vi "LVDT Setting.vi"(8 "error in (no error)":errorcluster) -> (0 "error out 2":errorcluster)   [LabVIEW 2015]
uses:
  Control Button/Save.ctl
  Control Button/Exit.ctl
  Control Button/Delete.ctl
  <vilib>/addons/database/Connection.llb/DB Tools Open Connec (String).vi
  <vilib>/addons/database/_DB Variant To Data/Database Variant To Data.xnode
  <vilib>/addons/database/NI_Database_API.lvlib
panel:
  in  "Delete":T1
  out "data":string[](array[string])
  out "Model change":string
  in  "Model Select":string(combo)
  out "error out":errorcluster
  in  "Exit":T2
  in  "Save":T3
  in  "Sensor Setting Data":T4 {"LVDT4Max(mm) AI3" format="%0.02f"; "LVDT3Max(mm) AI2" format="%0.02f"; "LVDT2Max(mm) AI1" format="%0.02f"; "LVDT1Max(mm) AI0" format="%0.02f"; "LVDT4Min(mm) AI3" format="%0.02f"; "LVDT3Min(mm) AI2" format="%0.02f"; "LVDT2Min(mm) AI1" format="%0.02f"; "LVDT1Min (mm)AI0" format="%0.02f"}
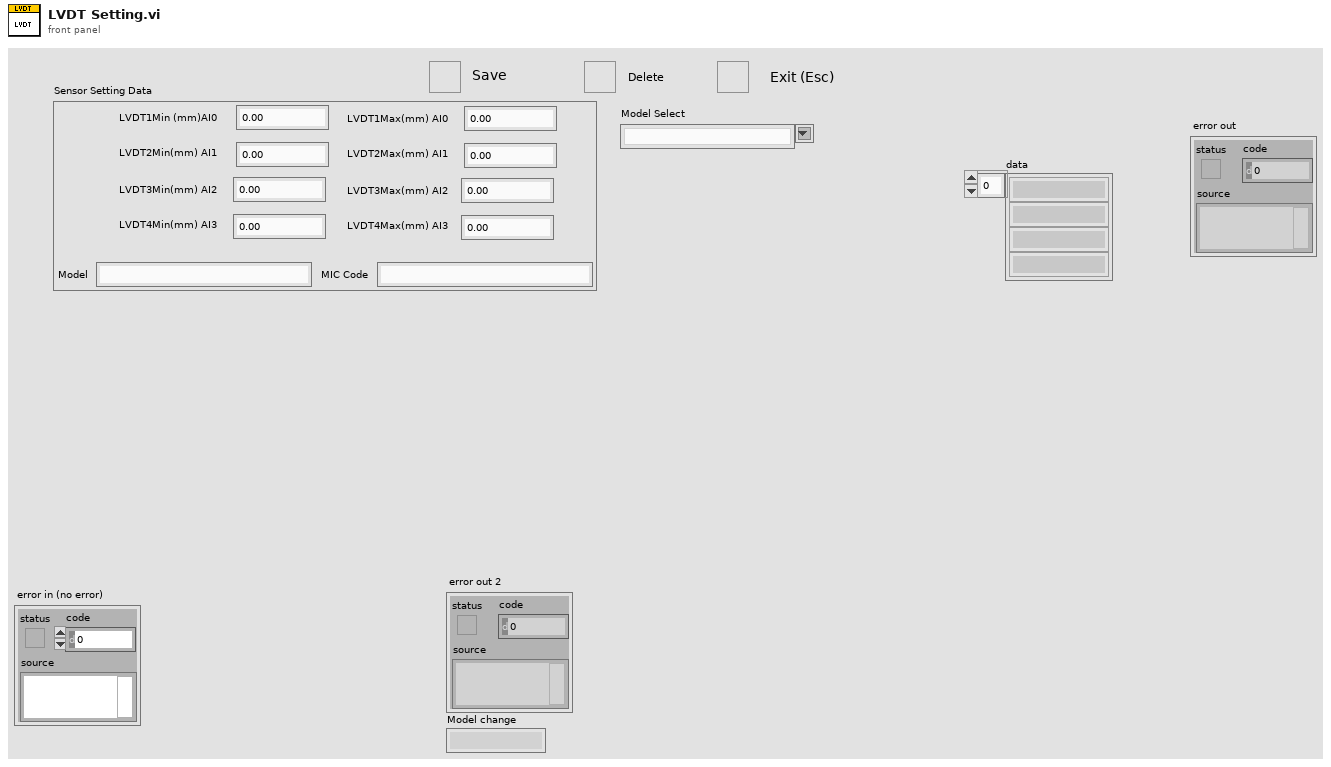
[diagram p1: front panel]
types:
  T1 = typedef "Delete.ctl" = bool
  T2 = typedef "Exit.ctl" = bool
  T3 = typedef "Save.ctl" = bool
  T4 = cluster{"LVDT1Max(mm) AI0":dbl, "LVDT1Min (mm)AI0":dbl, "LVDT2Max(mm) AI1":dbl, "LVDT2Min(mm) AI1":dbl, "LVDT3Max(mm) AI2":dbl, "LVDT3Min(mm) AI2":dbl, "LVDT4Max(mm) AI3":dbl, "LVDT4Min(mm) AI3":dbl, "Model":string, "MIC Code":string}
  T5 = typedef "NI_Database_API.lvlib/Conn ObjectReference.ctl" = refnum<k1>
  T6 = enum16{"Left Button", "Center Button", "Right Button", "Window Close"}
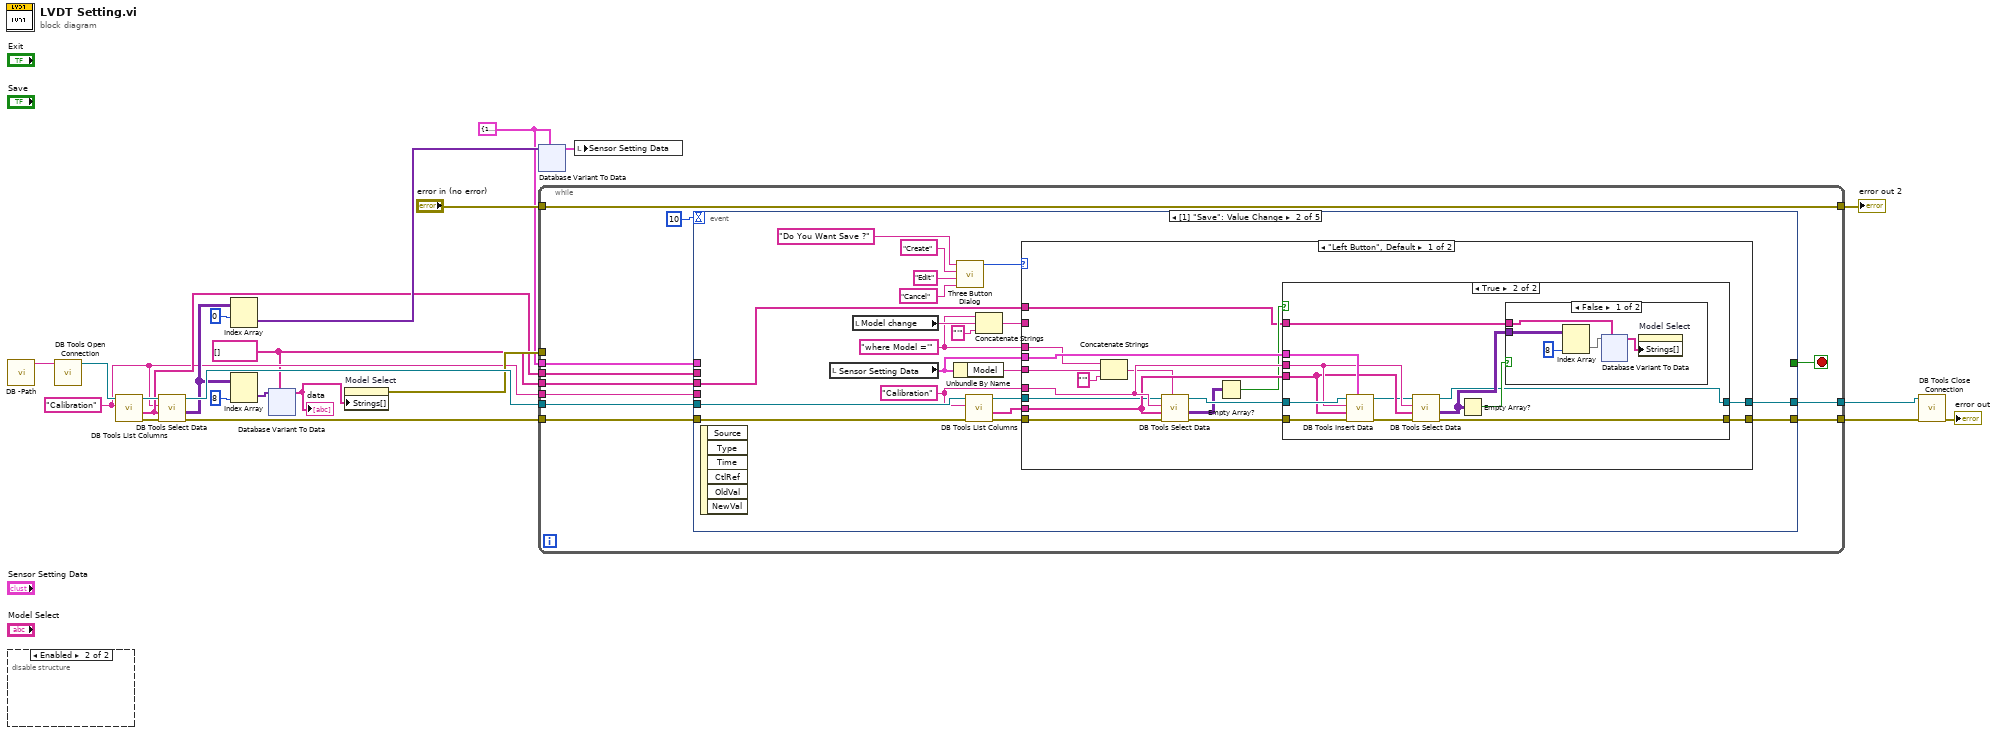
[diagram p0: block diagram]
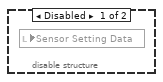
[diagram p2: hidden frame]
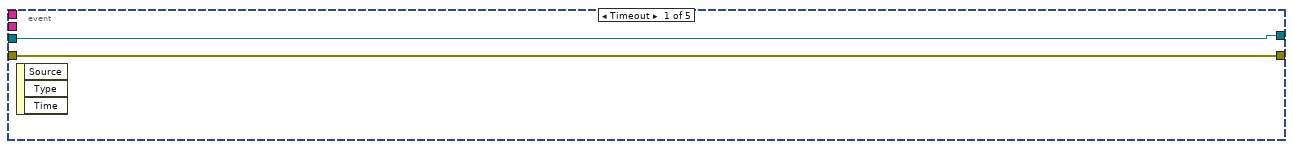
[diagram p3: hidden frame]
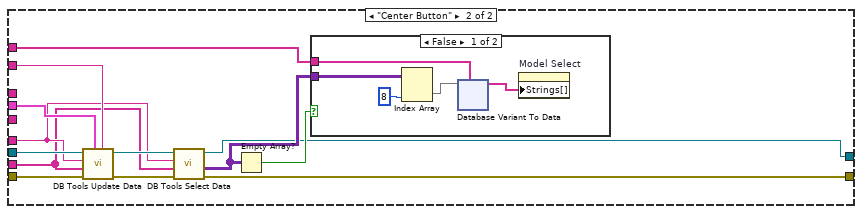
[diagram p6: hidden frame]
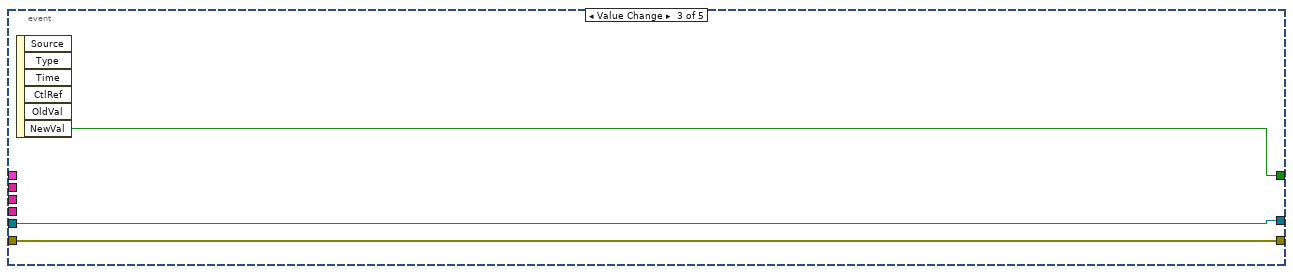
[diagram p8: hidden frame]
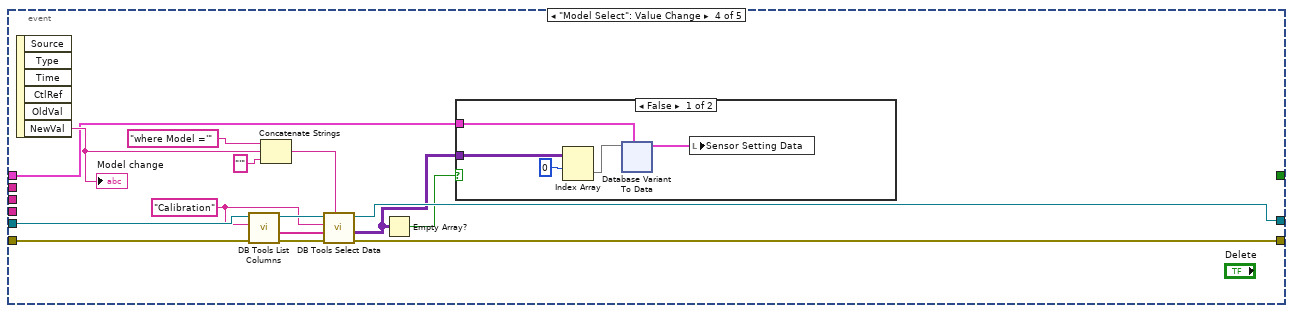
[diagram p9: hidden frame]
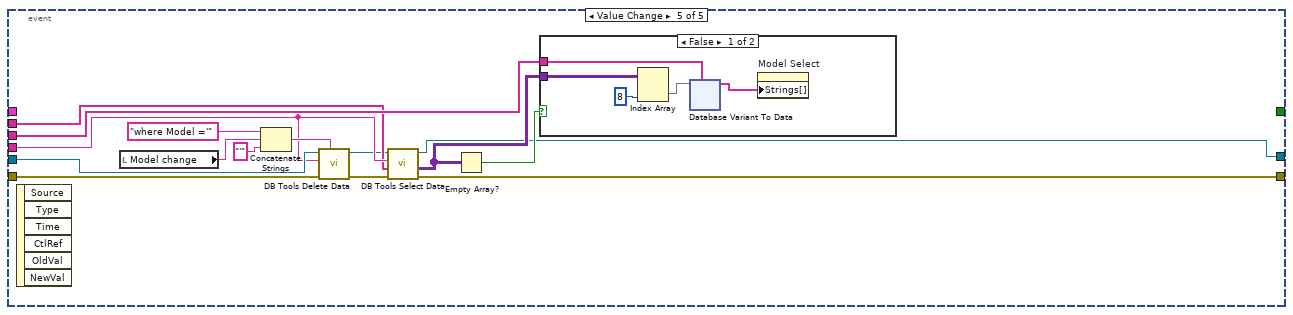
[diagram p11: hidden frame]
diagram:
  w1 = string[] [] ("Programlist")
  w9 = T4 {"LVDT1Max(mm) AI0"=10.0, "LVDT1Min (mm)AI0"=2.0, "LVDT2Max(mm) AI1"=10.0, "LVDT2Min(mm) AI1"=2.0, "LVDT3Max(mm) AI2"=10.0, "LVDT3Min(mm) AI2"=2.0, "LVDT4Max(mm) AI3"=10.0, "LVDT4Min(mm) AI3"=0.0, "Model"="", "MIC Code"=""} ("Sensor Setting Data")
  w2 = "Calibration" ("table")
  n1 = call "DB -Path.vi"() -> ("String"=w22:string)  [unwired: 11 in]
  n2 = disable-structure shown="Enabled" {
    frame Disabled {
      n3 = local read "Sensor Setting Data"() -> ()  [unwired: 1 in]
    }
    frame Enabled {
    }
  }
  n4 = call-poly <vilib>:"DB Tools Open Connection.vi"("connection information"=w22) -> ("connection reference"=w23:T5)  [unwired: 7 in, 1 out]
  n5 = call <vilib>:"DB Tools List Columns.vi"("table"=w2, "connection reference"=w23) -> ("error out"=w20:errorcluster, "columns"=w3:string[], "connection reference out"=w21:T5)  [unwired: 2 in, 1 out]
  n6 = call <vilib>:"DB Tools Select Data.vi"("error in (no error)"=w20, "columns"=w3, "table"=w2, "connection reference"=w21) -> ("error out"=w16:errorcluster, "data"=w6:variant[][], "connection reference out"=w17:T5)  [unwired: 2 in]
  n7 = Index Array(array=w6, index (row)=0) -> (element=w18:variant[])  [unwired: 1 in]
  n8 = Index Array(array=w6, index (col)=8 ("index (row)")) -> (element=w7:variant[])  [unwired: 1 in]
  n9 = xnode "Database Variant To Data"("database variant"=w7, "type"=w1) -> ("data"=w4:string[])  [unwired: 1 in, 1 out]
  "data" <- w4
  n10 = property on="Model Select" class="CmbBox"("Strings[]"=w4) -> (error out=w12:errorcluster)  [unwired: 2 in, 1 out]
  n11 = xnode "Database Variant To Data"("database variant"=w18, "type"=w9) -> ("data"=w8:T4)  [unwired: 1 in, 1 out]
  n12 = while {
    tunnel: w17 -> [w33]
    tunnel: w16 -> [w32]
    tunnel: [w31] -> w15
    tunnel: [w30] -> w14
    tunnel: w12 -> [_]
    tunnel: w9 -> [w28]
    tunnel: [w27] -> w10
    tunnel: "error in (no error)" -> [w27]
    tunnel: w3 -> [w26]
    tunnel: w2 -> [w25]
    tunnel: w1 -> [w24]
    stop <- w29 stop-if-true
    n13 = event shown="[1] \"Save\": Value Change" {
      selector: _ -> [_ _ _ _ _]
      dyn-events: _ -> [_ _ _ _ _]
      timeout: 10 -> [_ _ _ _ _]
      tunnel: w33 -> [w36 w51 w188 w198 w533]
      tunnel: w32 -> [w35 w50 w187 w197 w532]
      tunnel: [w36 w49 w188 w195 w525] -> w31
      tunnel: [w35 w48 w187 w196 w523] -> w30
      tunnel: [_ _ w186 _ _] -> w29
      tunnel: w28 -> [_ _ _ w191 _]
      tunnel: w26 -> [_ _ _ _ w527]
      tunnel: w25 -> [_ _ _ _ w528]
      tunnel: w24 -> [_ w40 _ _ w530]
      event Timeout {
        n14 = event-data() -> ()  [unwired: 1 in, 3 out]
      }
      event Value Change {
        w39 = "where Model ='"
        w47 = "Calibration" ("table")
        n15 = event-data() -> ()  [unwired: 1 in, 6 out]
        n16 = local read "Sensor Setting Data"() -> (w38:T4)
        n17 = local read "Model change"() -> (w44:string)
        n18 = Unbundle By Name(w38) -> ("Model"=w37:string)
        n19 = call <vilib>:"Three Button Dialog.vi"("Right Button Text (\"Cancel\")"="Cancel" ("Right Button Text (\"Cancel\")"), "Center Button Text (\"No\")"="Edit" ("F button name (\"Cancel\")"), "Left Button Text (\"Yes\")"="Create" ("T button name (\"OK\")"), "message"="Do You Want Save ?") -> ("Which Button?"=w56:T6)  [unwired: 7 in]
        n20 = call <vilib>:"DB Tools List Columns.vi"("error in (no error)"=w50, "table"=w47, "connection reference"=w51) -> ("error out"=w53:errorcluster, "columns"=w52:string[], "connection reference out"=w54:T5)  [unwired: 1 in, 1 out]
        n21 = Concatenate Strings(w39, w44, "'" ("string")) -> (w45:string)
        n22 = case shown="\"Left Button\", Default" w56 {
          tunnel: [w72 w135] -> w49
          tunnel: [w71 w133] -> w48
          tunnel: w54 -> [w67 w142]
          tunnel: w53 -> [w65 w141]
          tunnel: w52 -> [w68 w130]
          tunnel: w47 -> [w69 w131]
          tunnel: w38 -> [w70 w140]
          tunnel: w45 -> [_ w139]
          tunnel: w40 -> [w61 w132]
          tunnel: w39 -> [w60 _]
          tunnel: w37 -> [w59 _]
          frame "Left Button", Default {
            n23 = Concatenate Strings(w60, w59, "'" ("string")) -> (w57:string)
            n24 = call <vilib>:"DB Tools Select Data.vi"("condition"=w57, "error in (no error)"=w65, "columns"=w68, "table"=w69, "connection reference"=w67) -> ("error out"=w64:errorcluster, "data"=w63:variant[][], "connection reference out"=w66:T5)  [unwired: 1 in]
            n25 = Empty Array?(array=w63) -> (empty?=w62:bool)
            n26 = case shown="True" w62 {
              tunnel: w69 -> [_ w81]
              tunnel: w68 -> [_ w80]
              tunnel: w66 -> [w74 w86]
              tunnel: [w74 w78] -> w72
              tunnel: w64 -> [w73 w85]
              tunnel: [w73 w76] -> w71
              tunnel: w70 -> [_ w84]
              tunnel: w61 -> [_ w75]
              frame False {
              }
              frame True {
                n27 = call <vilib>:"DB Tools Insert Data.vi"("data"=w84, "error in (no error)"=w85, "columns"=w80, "table"=w81, "connection reference"=w86) -> ("error out"=w77:errorcluster, "connection reference out"=w79:T5)  [unwired: 5 in]
                n28 = call <vilib>:"DB Tools Select Data.vi"("error in (no error)"=w77, "columns"=w80, "table"=w81, "connection reference"=w79) -> ("error out"=w76:errorcluster, "data"=w83:variant[][], "connection reference out"=w78:T5)  [unwired: 2 in]
                n29 = Empty Array?(array=w83) -> (empty?=w82:bool)
                n30 = case shown="False" w82 {
                  tunnel: w83 -> [w90 _]
                  tunnel: w75 -> [w88 _]
                  frame False {
                    n31 = Index Array(array=w90, index (col)=8 ("disabled index (col)")) -> (element=w91:variant[])  [unwired: 1 in]
                    n32 = xnode "Database Variant To Data"("database variant"=w91, "type"=w88) -> ("data"=w87:string[])  [unwired: 1 in, 1 out]
                    n33 = property on="Model Select" class="CmbBox"("Strings[]"=w87) -> ()  [unwired: 2 in, 2 out]
                  }
                  frame True {
                  }
                }
              }
            }
          }
          frame "Center Button" {
            n34 = call <vilib>:"DB Tools Update Data.vi"("condition"=w139, "data"=w140, "error in (no error)"=w141, "columns"=w130, "table"=w131, "connection reference"=w142) -> ("error out"=w134:errorcluster, "connection reference out"=w136:T5)  [unwired: 4 in]
            n35 = call <vilib>:"DB Tools Select Data.vi"("error in (no error)"=w134, "columns"=w130, "table"=w131, "connection reference"=w136) -> ("error out"=w133:errorcluster, "data"=w137:variant[][], "connection reference out"=w135:T5)  [unwired: 2 in]
            n36 = Empty Array?(array=w137) -> (empty?=w138:bool)
            n37 = case shown="False" w138 {
              tunnel: w137 -> [w146 _]
              tunnel: w132 -> [w144 _]
              frame False {
                n38 = Index Array(array=w146, index (col)=8 ("disabled index (col)")) -> (element=w147:variant[])  [unwired: 1 in]
                n39 = xnode "Database Variant To Data"("database variant"=w147, "type"=w144) -> ("data"=w143:string[])  [unwired: 1 in, 1 out]
                n40 = property on="Model Select" class="CmbBox"("Strings[]"=w143) -> ()  [unwired: 2 in, 2 out]
              }
              frame True {
              }
            }
          }
        }
      }
      event Value Change {
        n41 = event-data() -> ("NewVal"=w186:T2)  [unwired: 1 in, 5 out]
      }
      event "Model Select": Value Change {
        w194 = "Calibration" ("table")
        n42 = event-data() -> ("NewVal"=w202:string)  [unwired: 1 in, 5 out]
        "Model change" <- w202
        n43 = call <vilib>:"DB Tools List Columns.vi"("error in (no error)"=w197, "table"=w194, "connection reference"=w198) -> ("error out"=w199:errorcluster, "columns"=w193:string[], "connection reference out"=w200:T5)  [unwired: 1 in, 1 out]
        n44 = Concatenate Strings("where Model ='", w202, "'" ("string")) -> (w192:string)
        n45 = call <vilib>:"DB Tools Select Data.vi"("condition"=w192, "error in (no error)"=w199, "columns"=w193, "table"=w194, "connection reference"=w200) -> ("error out"=w196:errorcluster, "data"=w190:variant[][], "connection reference out"=w195:T5)  [unwired: 1 in]
        n46 = Empty Array?(array=w190) -> (empty?=w189:bool)
        n47 = case shown="False" w189 {
          tunnel: w190 -> [w207 _]
          tunnel: w191 -> [w205 _]
          frame False {
            n48 = Index Array(array=w207, index (row)=0) -> (element=w206:variant[])  [unwired: 1 in]
            n49 = xnode "Database Variant To Data"("database variant"=w206, "type"=w205) -> ("data"=w204:T4)  [unwired: 1 in, 1 out]
            n50 = local write "Sensor Setting Data"(w204) -> ()
          }
          frame True {
          }
        }
      }
      event Value Change {
        n51 = event-data() -> ()  [unwired: 1 in, 6 out]
        n52 = local read "Model change"() -> (w537:string)
        n53 = Concatenate Strings("where Model ='", w537, "'" ("string")) -> (w534:string)
        n54 = call <vilib>:"DB Tools Delete Data.vi"("condition"=w534, "error in (no error)"=w532, "table"=w528, "connection reference"=w533) -> ("error out"=w524:errorcluster, "connection reference out"=w526:T5)  [unwired: 6 in]
        n55 = call <vilib>:"DB Tools Select Data.vi"("error in (no error)"=w524, "columns"=w527, "table"=w528, "connection reference"=w526) -> ("error out"=w523:errorcluster, "data"=w531:variant[][], "connection reference out"=w525:T5)  [unwired: 2 in]
        n56 = Empty Array?(array=w531) -> (empty?=w529:bool)
        n57 = case shown="False" w529 {
          tunnel: w531 -> [w541 _]
          tunnel: w530 -> [w539 _]
          frame False {
            n58 = Index Array(array=w541, index (col)=8 ("disabled index (col)")) -> (element=w542:variant[])  [unwired: 1 in]
            n59 = xnode "Database Variant To Data"("database variant"=w542, "type"=w539) -> ("data"=w538:string[])  [unwired: 1 in, 1 out]
            n60 = property on="Model Select" class="CmbBox"("Strings[]"=w538) -> ()  [unwired: 2 in, 2 out]
          }
          frame True {
          }
        }
      }
    }
  }
  "error out 2" <- w10
  n61 = local write "Sensor Setting Data"(w8) -> ()
  n62 = call <vilib>:"DB Tools Close Connection.vi"("error in (no error)"=w14, "connection reference"=w15) -> ("error out"=→"error out":errorcluster)  [unwired: 5 in]
